vi "Actor Core.vi"(8 "error in":errorcluster, 11 "Power Meter Display in":refnum<class "Power Meter Display.lvclass">) -> (0 "error out":errorcluster, 3 "Actor out":refnum<class "Actor.lvclass">)   [LabVIEW 2012, in "Display Panel.lvlib" / "Power Meter Display.lvclass"]
doc: "(<B>Filename</B>: Actor Framework.lvlib:Actor.lvclass:Actor Core.vi)\n\nReceives messages to the actor, reacts to them, and initiates any error handling that may shut the actor down.\n\nDescendant classes may override this VI to append parallel tasks for the actor to complete while it handles messages. Overrides use the Call Parent Method node."
uses:
  Power Meter Display.lvclass
  <vilib>/ActorFramework/Actor/Actor.lvclass
  Power Meter Display.lvclass/Power Meter Display.ctl
  Abstract Display/Abstract Display.lvclass/Abstract Display.ctl
  Abstract Display/Abstract Display.lvclass
  <vilib>/ActorFramework/Actor/Actor.lvclass/Actor.ctl
  <vilib>/ActorFramework/Message Enqueuer/Message Enqueuer.lvclass/Message Enqueuer.ctl
  1600Card/1600 Card Actor Messages/Write data Stop Bit Msg/Write data Stop Bit Msg.lvclass/Write data Stop Bit Msg.ctl
  <vilib>/ActorFramework/Message Enqueuer/Enqueue.vi
  <vilib>/ActorFramework/Message Enqueuer/Init from Existing Queue.vi
  <vilib>/ActorFramework/Message Priority Queue/Priority Enqueue.vi
  <vilib>/ActorFramework/Message Enqueuer/Message Enqueuer.lvclass
  1600Card/1600 Card Actor Messages/Write data Stop Bit Msg/Write data Stop Bit Msg.lvclass
  <vilib>/ActorFramework/Stop Msg/Stop Msg.lvclass
  Display Panel.lvlib
panel:
  in  "Caption.Text":string
  in  "blink?":bool
  out "Numeric Control 2":i32
  out "Start blinking":bool=TRUE
  out "Numeric Control":i32
  out "Blinker":bool caption="Warming"
  in  "EXit":bool
  in  "Stop":bool
  out "Time":dbl format="%<%H:%M:%S>t"
  out "Watt-Hour":dbl
  out "Frequency":dbl
  out "Power":dbl
  out "Current":dbl
  out "Voltage":dbl
  out "Card #":dbl
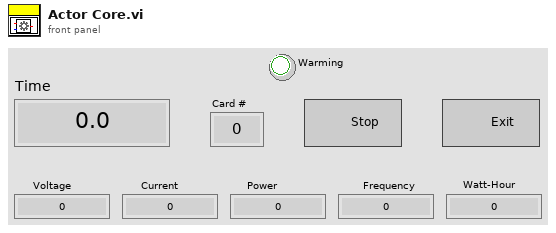
[diagram p1: front panel]
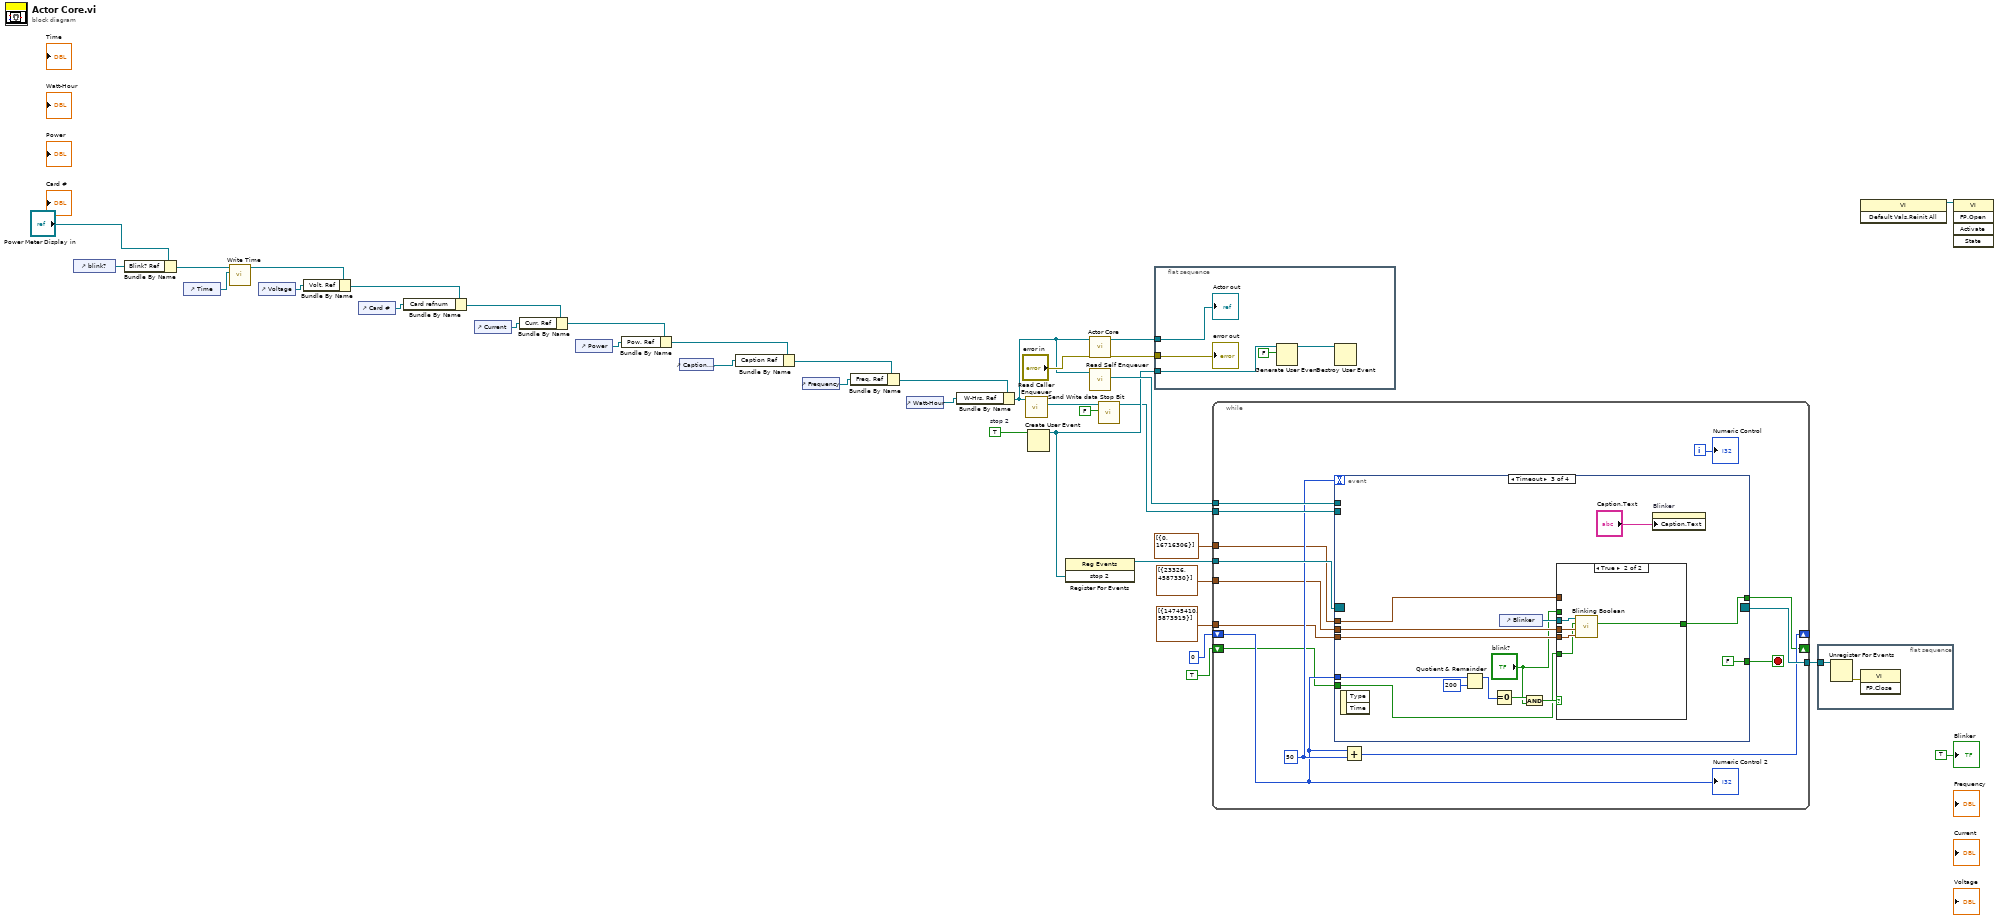
[diagram p0: block diagram]
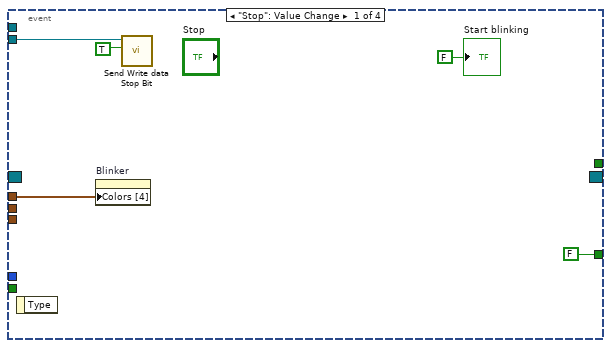
[diagram p2: hidden frame]
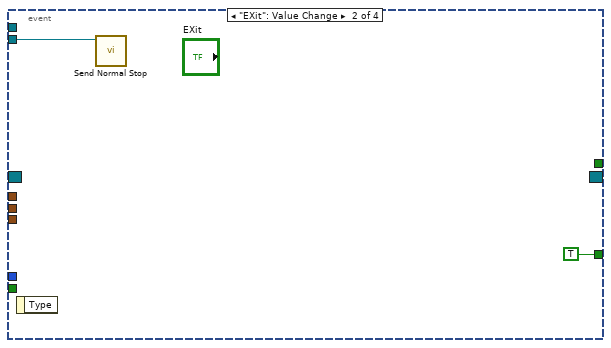
[diagram p3: hidden frame]
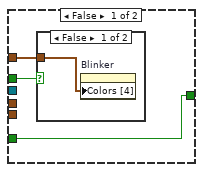
[diagram p4: hidden frame]
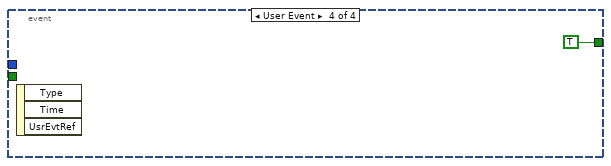
[diagram p6: hidden frame]
diagram:
  w15 = TRUE  # stop 2
  n1 = control-ref of="blink?"() -> (w7:refnum<vi>)
  n2 = Bundle By Name(cluster="Power Meter Display in", "Blink? Ref"=w7) -> (w8:refnum<class "Power Meter Display.lvclass">)
  n3 = control-ref of="Time"() -> (w23:refnum<vi>)
  n4 = call "Write Time.vi"("Time"=w23, "Abstract Display in"=w8) -> ("Abstract Display out"=w24:refnum<class "Power Meter Display.lvclass">)  [unwired: 8 in, 1 out]
  n5 = control-ref of="Voltage"() -> (w35:refnum<vi>)
  n6 = Bundle By Name(cluster=w24, "Volt. Ref"=w35) -> (w33:refnum<class "Power Meter Display.lvclass">)
  n7 = control-ref of="Card #"() -> (w32:refnum<vi>)
  n8 = Bundle By Name(cluster=w33, "Card refnum"=w32) -> (w31:refnum<class "Power Meter Display.lvclass">)
  n9 = control-ref of="Current"() -> (w28:refnum<vi>)
  n10 = Bundle By Name(cluster=w31, "Curr. Ref"=w28) -> (w30:refnum<class "Power Meter Display.lvclass">)
  n11 = control-ref of="Power"() -> (w27:refnum<vi>)
  n12 = Bundle By Name(cluster=w30, "Pow. Ref"=w27) -> (w3:refnum<class "Power Meter Display.lvclass">)
  n13 = control-ref of="Caption.Text"() -> (w1:refnum<vi>)
  n14 = Bundle By Name(cluster=w3, "Caption Ref"=w1) -> (w2:refnum<class "Power Meter Display.lvclass">)
  n15 = control-ref of="Frequency"() -> (w26:refnum<vi>)
  n16 = Bundle By Name(cluster=w2, "Freq. Ref"=w26) -> (w29:refnum<class "Power Meter Display.lvclass">)
  n17 = control-ref of="Watt-Hour"() -> (w25:refnum<vi>)
  n18 = Bundle By Name(cluster=w29, "W-Hrs. Ref"=w25) -> (w20:refnum<class "Power Meter Display.lvclass">)
  n19 = call <vilib>:"Read Caller Enqueuer.vi"("Actor"=w20) -> ("Caller Enqueuer"=w13:refnum<class "Message Enqueuer.lvclass">)  [unwired: 10 in]
  n20 = Create User Event(user event datatype=w15) -> (user event=w16:refnum<user-event>)  [unwired: 1 in, 1 out]
  n21 = register-events(w16) -> (reference out=w18:refnum<event-registration>)  [unwired: 2 in, 1 out]
  n22 = call-parent "Actor Core.vi"("error in"="error in", "Abstract Display in"=w20) -> ("error out"=w37:errorcluster, "Actor out"=w36:refnum<class "Actor.lvclass">)  [unwired: 8 in]
  n23 = call <vilib>:"Read Self Enqueuer.vi"("Actor"=w20) -> ("Self Enqueuer"=w22:refnum<class "Message Enqueuer.lvclass">)  [unwired: 10 in]
  n24 = call "Send Write data Stop Bit.vi"("stop bit"=FALSE, "Message Enqueuer"=w13) -> ("Message Enqueuer out"=w12:refnum<class "Message Enqueuer.lvclass">)  [unwired: 8 in, 1 out]
  n25 = flat-sequence {
    tunnel: w37 -> [w42]
    tunnel: w36 -> [w41]
    tunnel: w16 -> [w40]
    frame #0 {
      n26 = Generate User Event(user event=w40, event data cluster=FALSE ("event data")) -> (user event out=w38:refnum<user-event>)  [unwired: 1 in, 1 out]
      n27 = Destroy User Event(user event=w38) -> ()  [unwired: 1 in, 1 out]
      "error out" <- w42
      "Actor out" <- w41
    }
  }
  n28 = while {
    tunnel: w22 -> [w56]
    tunnel: w12 -> [w54]
    tunnel: cluster{u32, u32}[] [{0, 16716306}] ("Colors [4]") -> [w47]
    tunnel: w18 -> [w53]
    tunnel: [w52] -> w17
    shift-right: [w49] -> _
    shift-left: 0 -> [w48]
    tunnel: cluster{u32, u32}[] [{14745410, 5873919}] ("Colors [4]") -> [w46]
    shift-right: [w43] -> _
    shift-left: TRUE -> [w44]
    tunnel: cluster{u32, u32}[] [{23326, 4587330}] ("Color 2 (Background, Foreground)") -> [w45]
    i -> [w51]
    stop <- w55 stop-if-true
    w50 = 50
    n29 = event shown="[2] Timeout" {
      selector: w53 -> [_ _ _ _]
      dyn-events: [_ _ _ _] -> w52
      timeout: w50 -> [_ _ _ _]
      tunnel: w56 -> [_ _ _ _]
      tunnel: [FALSE TRUE FALSE TRUE] -> w55
      tunnel: w54 -> [w59 w62 _ _]
      tunnel: w47 -> [w61 _ w66 _]
      tunnel: w48 -> [_ _ w75 _]
      tunnel: w46 -> [_ _ w71 _]
      tunnel: w45 -> [_ _ w70 _]
      tunnel: w44 -> [_ _ w68 _]
      tunnel: [_ _ w67 _] -> w43
      event "Stop": Value Change {
        n30 = event-data() -> ()  [unwired: 1 in, 1 out]
        n31 = property on="Blinker" class="Bool (strict)"("Colors [4]"=w61) -> ()  [unwired: 2 in, 2 out]
        n32 = call "Send Write data Stop Bit.vi"("stop bit"=TRUE, "Message Enqueuer"=w59) -> ()  [unwired: 8 in, 2 out]
        "Start blinking" <- FALSE ("stop blinking")
      }
      event "EXit": Value Change {
        n33 = event-data() -> ()  [unwired: 1 in, 1 out]
        n34 = call <vilib>:"Send Normal Stop.vi"("Message Enqueuer"=w62) -> ()  [unwired: 10 in, 1 out]
      }
      event Timeout {
        n35 = event-data() -> ()  [unwired: 1 in, 2 out]
        n36 = Quotient & Remainder(x=w75, y=200) -> (x-y*floor(x/y)=w74:i32)  [unwired: 1 out]
        n37 = Equal To 0?(x=w74) -> (x = 0?=w73:bool)
        n38 = control-ref of="Blinker"() -> (w69:refnum<vi>)
        n39 = And(x=w73, y="blink?") -> (x .and. y?=w72:bool)
        n40 = case shown="True" w72 {
          tunnel: w71 -> [_ w86]
          tunnel: w70 -> [_ w85]
          tunnel: w69 -> [_ w84]
          tunnel: w68 -> [w80 w83]
          tunnel: [w80 w82] -> w67
          tunnel: w66 -> [w78 _]
          tunnel: "blink?" -> [w79 _]
          frame False {
            n41 = case shown="False" w79 {
              tunnel: w78 -> [w81 _]
              frame False {
                n42 = property on="Blinker" class="Bool (strict)"("Colors [4]"=w81) -> ()  [unwired: 2 in, 2 out]
              }
              frame True {
              }
            }
          }
          frame True {
            n43 = call "Blinking Boolean.vi"("Color 2 (Background, Foreground)"=w86, "Color 1 (Background, Foreground)"=w85, "Shift in"=w83, "Bool Refnum"=w84) -> ("Shift out"=w82:bool)  [unwired: 7 in]
          }
        }
        n44 = property on="Blinker" class="Bool (strict)"("Caption.Text"="Caption.Text") -> ()  [unwired: 2 in, 2 out]
      }
      event User Event {
        n45 = event-data() -> ()  [unwired: 1 in, 3 out]
      }
    }
    n46 = Add(x=w48, y=w50) -> (x+y=w49:i32)
    "Numeric Control" <- w51
    "Numeric Control 2" <- w48
  }
  n47 = flat-sequence {
    tunnel: w17 -> [w89]
    frame #0 {
      n48 = Unregister For Events(event registration refnum=w89) -> (error out=w88:errorcluster)  [unwired: 1 in]
      n49 = invoke class="VI" method="FP.Close"(error in=w88) -> ()  [unwired: 2 in, 3 out]
    }
  }
  n50 = invoke class="VI" method="Default Vals.Reinit All"() -> (reference out=w21:refnum<vi>)  [unwired: 3 in, 2 out]
  n51 = invoke class="VI" method="FP.Open"(reference=w21) -> ()  [unwired: 4 in, 5 out]
  "Blinker" <- TRUE ("Boolean")
